vi "Data Socket mio writer.vi"(1 "stop":bool, 2 "String":string) -> (0 "Indicatore":dbl)   [LabVIEW 2012]
panel:
  out "Stringa\nconcatenata":string
  # "Ricordarsi di avviare DataSocket Server"
  # "Default:\n\nlocalhost/samplenum"
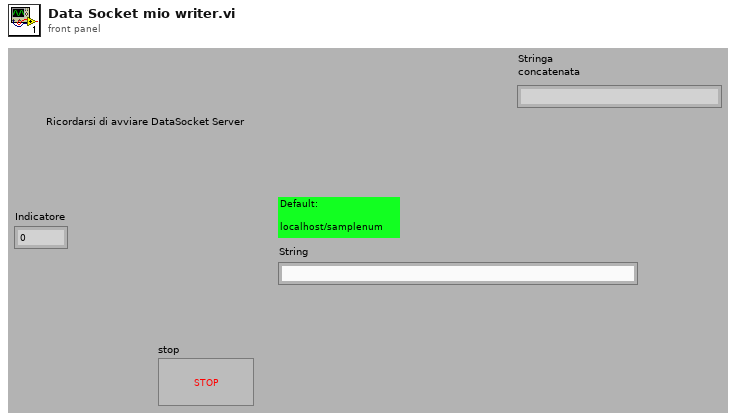
[diagram p1: front panel]
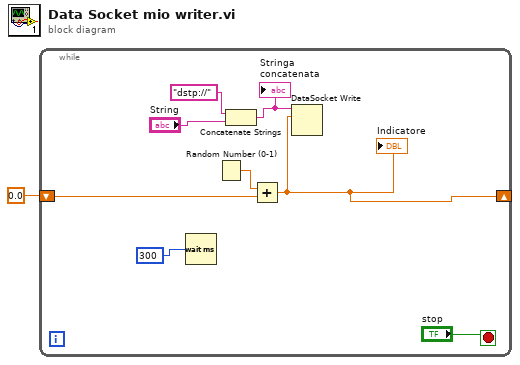
[diagram p0: block diagram]
diagram:
  n1 = while {
    shift-right: [w6] -> _
    shift-left: 0.0 -> [w7]
    stop <- "stop" stop-if-true
    n2 = Wait (ms)(milliseconds to wait=u32 300) -> ()  [unwired: 1 out]
    n3 = Random Number (0-1)() -> (number: 0 to 1=w8:dbl)
    n4 = Concatenate Strings("dstp://" ("URL"), "String") -> (w3:string)
    "Stringa\nconcatenata" <- w3
    n5 = Add(x=w8, y=w7) -> (x+y=w6:dbl)
    "Indicatore" <- w6
    n6 = DataSocket Write(10:w6, 11:w3) -> ()  [unwired: 2 in, 3 out]
  }
